vi "clusters.vi"() -> ()   [LabVIEW 2023]
panel:
  out "Warning Text":string
  out "WARNING?":bool
  out "Min Temp":dbl
  out "Max Temp":dbl
  out "Current Temp":dbl
  in  "Weather Data In":T1
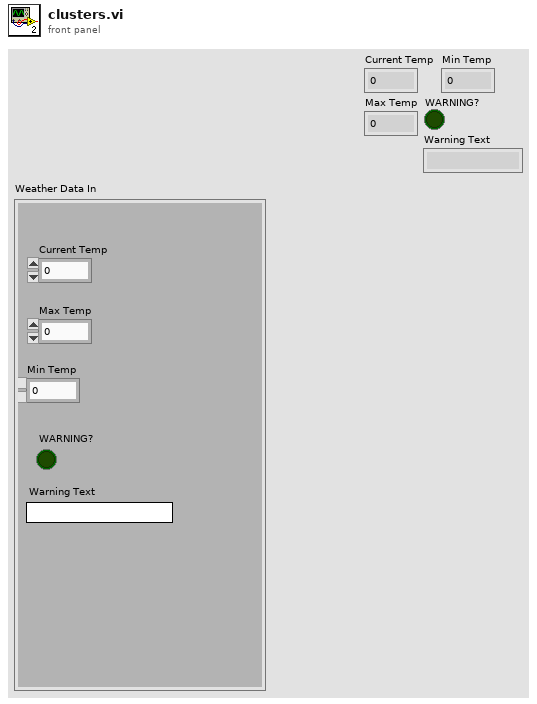
[diagram p1: front panel]
types:
  T1 = cluster{"Current Temp":dbl, "Max Temp":dbl, "Min Temp":dbl, "WARNING?\n":bool, "Warning Text":string}
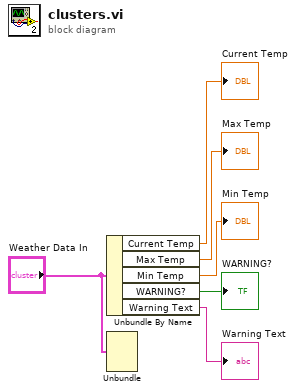
[diagram p0: block diagram]
diagram:
  n1 = Unbundle By Name("Weather Data In") -> ("Current Temp"=→"Current Temp":dbl, "Max Temp"=→"Max Temp":dbl, "Min Temp"=→"Min Temp":dbl, "WARNING?"=→"WARNING?":bool, "Warning Text"=→"Warning Text":string)
  n2 = Unbundle("Weather Data In") -> ()  [unwired: 5 out]
